vi "Mischer_preassure_readout.vi"(7 "Gauge Number (1)":T1) -> (1 "Reading [V/mbar]":dbl)   [LabVIEW 2019]
uses:
  Mischer/BOC Edwards TIC/Turbo Instrument Controller.llb/Type Def - Gauge Num Selection.ctl
  Instrument_Setup.vi
panel:
  out "error out":errorcluster caption="Fehler (Ausgang)"
  out "Gauge Name 1":string
  in  "error in (no error)":errorcluster caption="Fehler (Eingang, kein Fehler)"
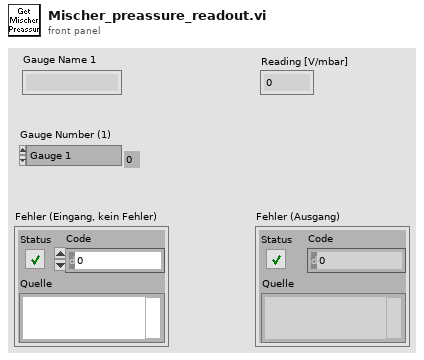
[diagram p1: front panel]
types:
  T1 = typedef "Type Def - Gauge Num Selection.ctl" = enum16{"Gauge 1", "Gauge 2", "Gauge 3", "Gauge 4", "Gauge 5", "Gauge 6"}
  T2 = cluster{"Arduino Levelmeter":refnum<visa-resource-name>, "TIC Comport":refnum<visa-resource-name>}
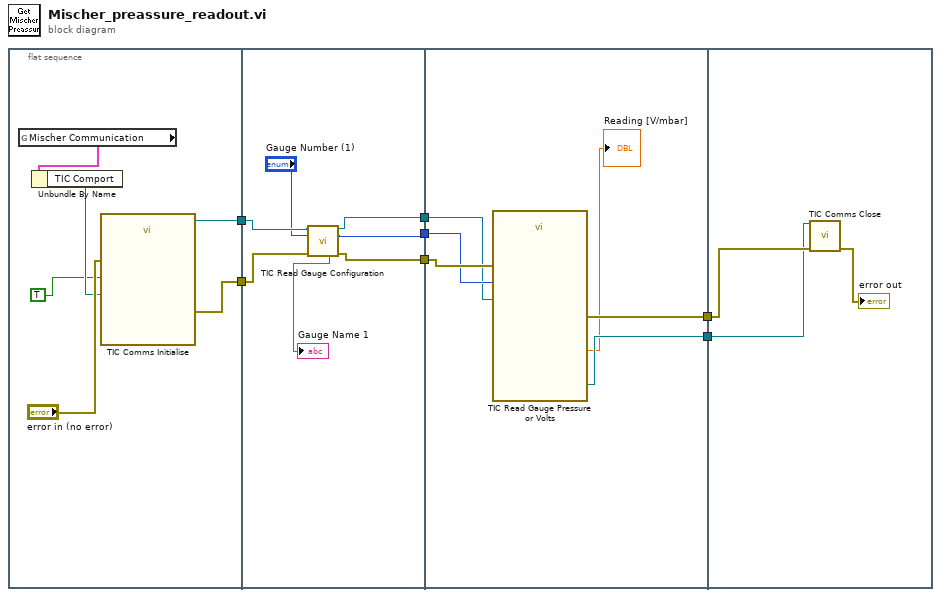
[diagram p0: block diagram]
diagram:
  n1 = flat-sequence {
    tunnel: [w10] -> w7
    tunnel: [w8] -> w6
    tunnel: w7 -> [w20]
    tunnel: w6 -> [w15]
    tunnel: [w17] -> w5
    tunnel: [w16] -> w4
    tunnel: [w18] -> w3
    tunnel: w5 -> [w25]
    tunnel: w4 -> [w26]
    tunnel: w3 -> [w24]
    tunnel: [w23] -> w2
    tunnel: [w22] -> w1
    tunnel: w2 -> [w29]
    tunnel: w1 -> [w28]
    frame #0 {
      n2 = global read "Instrument_Setup.vi" "Mischer Communication"() -> (w12:T2)
      n3 = Unbundle By Name(w12) -> ("TIC Comport"=w11:refnum<visa-resource-name>)
      n4 = call "TIC Comms Initialise.vi"("VISA Resource Name"=w11, "ID Query (T: Check)"=TRUE, "error in (no error)"="error in (no error)") -> ("VISA session (Dup)"=w10:refnum<visa-resource-name>, "error out"=w8:errorcluster)  [unwired: 11 in]
    }
    frame #1 {
      n5 = call "TIC Read Gauge Configuration.vi"("VISA Session In"=w20, "Gauge Number (1)"="Gauge Number (1)", "error in (no error)"=w15) -> ("VISA Session (Dup)"=w18:refnum<visa-resource-name>, "Gauge Number (Dup)"=w17:T1, "User Gauge Name"=→"Gauge Name 1":string, "error out"=w16:errorcluster)  [unwired: 7 in, 2 out]
    }
    frame #2 {
      n6 = call "TIC Read Gauge Pressure or Volts.vi"("VISA Session In"=w24, "Gauge Number (1)"=w25, "error in (no error)"=w26) -> ("VISA Session (Dup)"=w22:refnum<visa-resource-name>, "Reading"=→"Reading [V/mbar]":dbl, "error out"=w23:errorcluster)  [unwired: 8 in, 2 out]
    }
    frame #3 {
      n7 = call "TIC Comms Close.vi"("VISA Resource Name"=w28, "error in (no error)"=w29) -> ("error out"=→"error out":errorcluster)  [unwired: 13 in]
    }
  }
